vi "Generate Zernike Vectors.vi"(6 "error in (no error)":errorcluster, 9 "Automation State in":T1={"Automation State"=enum."Idle", "Handle out"=0, "ZO State"={"ZO Settings"={"Acquisition Settings"={"Save?"=FALSE, "DCIMG Path"=path "", "Filename"="", "Total Frames"=0, "Sender"=enum."UI"}, "Shift Amplitude"=0.0, "Initial Zernike Vector"=[]}, "Zernike Size"=15, "Points per order"=15, "Zernike State"=enum."Idle", "Zernike Vectors"=[], "Total Frames"=15, "Current Frame"=15}, "Zstack State"={"Zstack Settings"={"Acquisition Settings"={"Save?"=FALSE, "DCIMG Path"=path "", "Filename"="", "Total Frames"=0, "Sender"=enum."UI"}, "XYZ start"=[], "XYZ end"=[]}, "Zstack State"=enum."Idle", "Stack Coordinates"=[], "Total Frames"=15, "Current Frame"=15}}) -> (0 "error out":errorcluster, 3 "Automation State Out":T1={"Automation State"=enum."Idle", "Handle out"=0, "ZO State"={"ZO Settings"={"Acquisition Settings"={"Save?"=FALSE, "DCIMG Path"=path "", "Filename"="", "Total Frames"=0, "Sender"=enum."UI"}, "Shift Amplitude"=0.0, "Initial Zernike Vector"=[]}, "Zernike Size"=15, "Points per order"=15, "Zernike State"=enum."Idle", "Zernike Vectors"=[], "Total Frames"=15, "Current Frame"=15}, "Zstack State"={"Zstack Settings"={"Acquisition Settings"={"Save?"=FALSE, "DCIMG Path"=path "", "Filename"="", "Total Frames"=0, "Sender"=enum."UI"}, "XYZ start"=[], "XYZ end"=[]}, "Zstack State"=enum."Idle", "Stack Coordinates"=[], "Total Frames"=15, "Current Frame"=15}})   [LabVIEW 2015, in "Automation.lvlib"]
uses:
  Automation.lvlib
  Automation State.ctl
  Automation Loop State.ctl
  ZO State.ctl
  ZO Settings.ctl
  Camera/Acquisition Settings.ctl
  Zstack State.ctl
  Zstack Settings.ctl
  Camera/Camera.lvlib
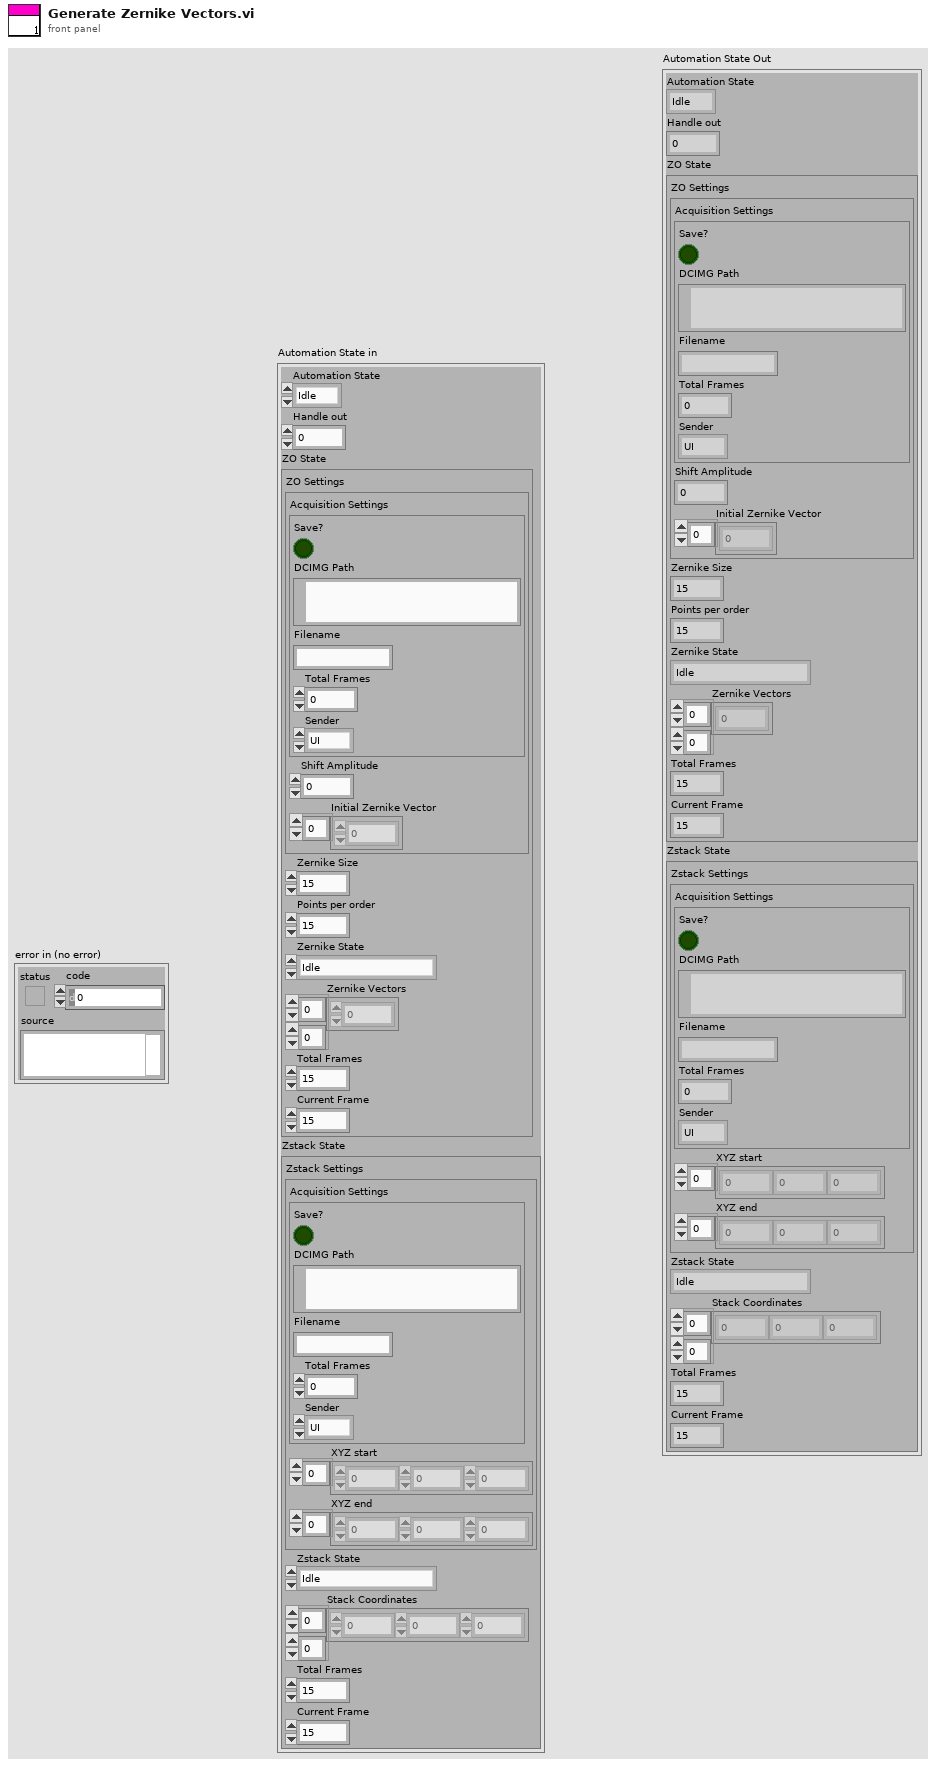
[diagram p1: front panel]
types:
  T1 = typedef "Automation.lvlib/Automation State.ctl" = cluster{"Automation State":T2, "Handle out":u32, "ZO State":T3, "Zstack State":T6}
  T2 = typedef "Automation.lvlib/Automation Loop State.ctl" = enum16{"Idle", "Zernike Optimization", "Z Stack"}
  T3 = typedef "Automation.lvlib/ZO State.ctl" = cluster{"ZO Settings":T4, "Zernike Size":i32, "Points per order":i32, "Zernike State":enum16{"Idle", "Waiting for Camera Init.", "Wait for camera frame", "Ready for new mirror config"}, "Zernike Vectors":dbl[][], "Total Frames":i32, "Current Frame":i32}
  T4 = typedef "Automation.lvlib/ZO Settings.ctl" = cluster{"Acquisition Settings":T5, "Shift Amplitude":dbl, "Initial Zernike Vector":dbl[]}
  T5 = typedef "Camera.lvlib/Acquisition Settings.ctl" = cluster{"Save?":bool, "DCIMG Path":path, "Filename":string, "Total Frames":i32, "Sender":enum16{"UI", "Automation"}}
  T6 = typedef "Automation.lvlib/Zstack State.ctl" = cluster{"Zstack Settings":T7, "Zstack State":enum16{"Idle", "Waiting for Camera Init.", "Wait for camera frame", "Ready for new position"}, "Stack Coordinates":dbl[][], "Total Frames":i32, "Current Frame":i32}
  T7 = typedef "Automation.lvlib/Zstack Settings.ctl" = cluster{"Acquisition Settings":T5, "XYZ start":dbl[], "XYZ end":dbl[]}
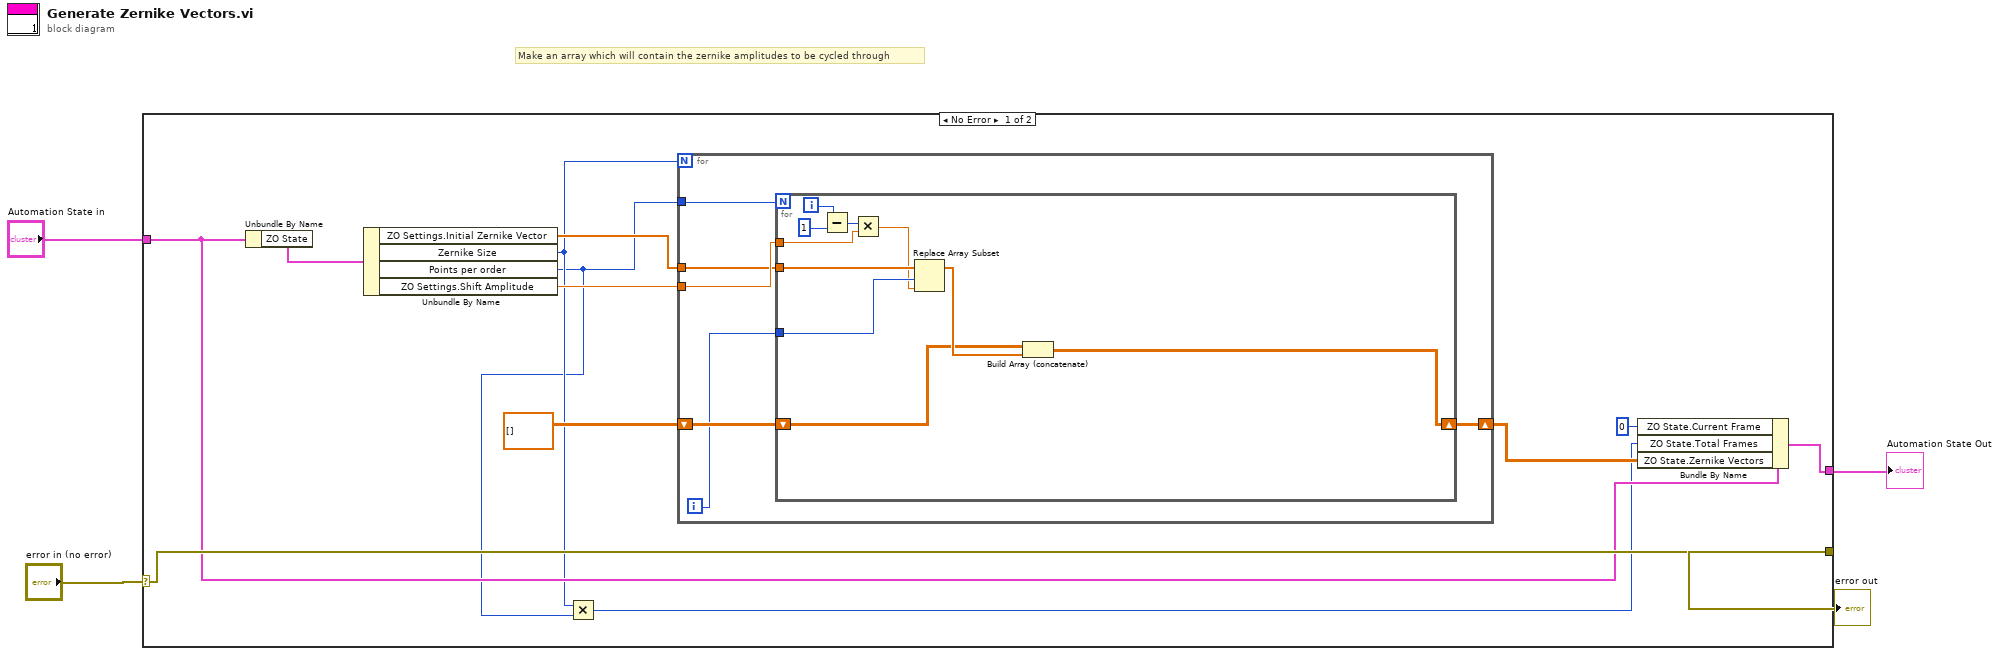
[diagram p0: block diagram]
diagram:
  # "Make an array which will contain the zernike amplitudes to be cycled through"
  n1 = case shown="No Error" "error in (no error)" {
    selector: "error in (no error)" -> [w16 w34]
    tunnel: [w16 w34] -> w3
    tunnel: "Automation State in" -> [w11 w33]
    tunnel: [w9 w33] -> w1
    frame No Error {
      n2 = Unbundle By Name(w11) -> ("ZO State"=w15:T3)
      n3 = Unbundle By Name(w15) -> ("ZO Settings.Initial Zernike Vector"=w12:dbl[], "Zernike Size"=w8:i32, "Points per order"=w7:i32, "ZO Settings.Shift Amplitude"=w14:dbl)
      n4 = Multiply(x=w8, y=w7) -> (x*y=w6:i32)
      n5 = for {
        N: w8 -> [_]
        tunnel: w7 -> [w22]
        tunnel: w14 -> [w21]
        shift-right: [w17] -> w10
        shift-left: dbl[][] [] ("ZO Settings.Initial Zernike Vector") -> [w20]
        tunnel: w12 -> [w19]
        i -> [w18]
        n6 = for {
          N: w22 -> [_]
          tunnel: w21 -> [w30]
          shift-right: [w23] -> w17
          shift-left: w20 -> [w24]
          tunnel: w19 -> [w28]
          tunnel: w18 -> [w27]
          i -> [w29]
          n7 = Subtract(x=w29, y=1) -> (x-y=w31:i32)
          n8 = Multiply(x=w31, y=w30) -> (x*y=w26:dbl)
          n9 = Replace Array Subset(array=w28, new element=w26, index=w27) -> (w25:dbl[])
          n10 = Build Array (concatenate)(w24, w25) -> (w23:dbl[][])
        }
      }
      n11 = Bundle By Name(cluster=w11, "ZO State.Current Frame"=0, "ZO State.Total Frames"=w6, "ZO State.Zernike Vectors"=w10) -> (w9:T1)
    }
    frame Error {
    }
  }
  "error out" <- w3
  "Automation State Out" <- w1
